vi "Evaluate Checksum.vi"(5 "Parallel in":refnum<class "Parallel.lvclass">, 6 "Path Builder":refnum<class "IPath Builder.lvclass">, 7 "Linked List ID":string, 8 "error in (no error)":errorcluster, 11 "Linked List Ref":refnum<data-value>) -> (0 "error out":errorcluster, 1 "Checksums Match":bool, 2 "Paths":path[](array[path]), 3 "Linked List Ref out":refnum<data-value>)   [LabVIEW 2017]
uses:
  linked-list/Source/Linked List/Linked List Ref/Linked List Ref.lvclass
  Parallel.lvclass
  linked-list/Source/Linked List/ILinkedList/ILinked List.lvclass
  Path Builder/IPath Builder/IPath Builder.lvclass
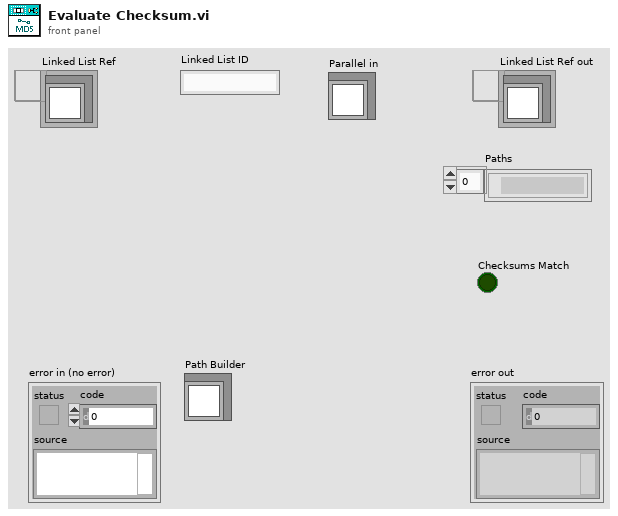
[diagram p1: front panel]
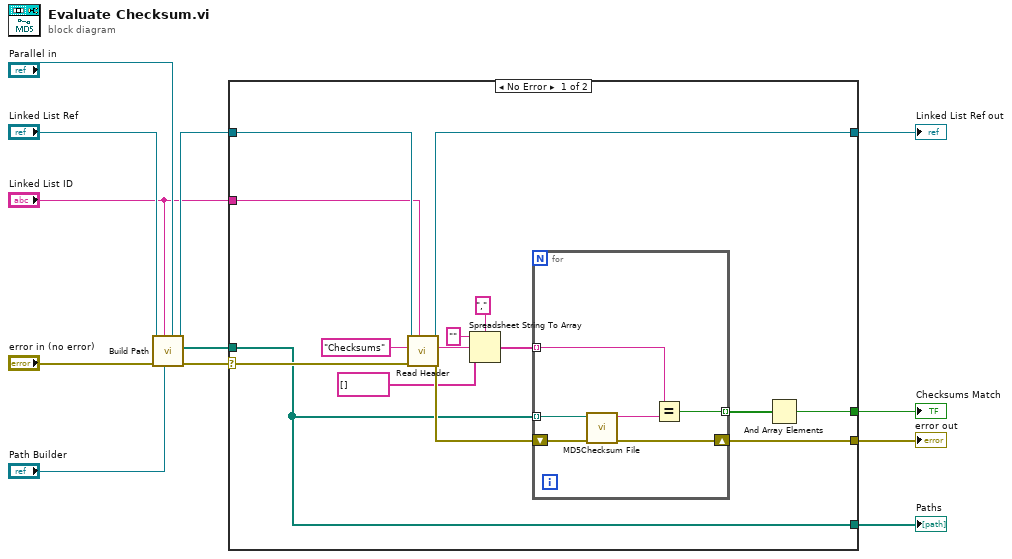
[diagram p0: block diagram]
diagram:
  n1 = call-dynamic "Build Path.vi"("Parallel in"="Parallel in", "Path Builder"="Path Builder", "Linked List ID"="Linked List ID", "error in (no error)"="error in (no error)", "Linked List Ref"="Linked List Ref") -> ("error out"=w5:errorcluster, "Paths"=w4:path[], "Linked List Ref out"=w8:refnum<data-value>)  [unwired: 4 in]
  n2 = case shown="No Error" w5 {
    selector: w5 -> [w20 w34]
    tunnel: [w18 _] -> w2
    tunnel: [w25 w35] -> w7
    tunnel: [w23 w34] -> w3
    tunnel: w8 -> [w22 w35]
    tunnel: "Linked List ID" -> [w21 _]
    tunnel: w4 -> [w19 _]
    tunnel: [w19 _] -> w1
    frame No Error {
      n3 = call "Read Header.vi"("Linked List ID"=w21, "error in (no error)"=w20, "Header Name"="Checksums", "Linked List Ref"=w22) -> ("error out"=w24:errorcluster, "Header Value"=w17:string, "Linked List Ref out"=w25:refnum<data-value>)  [unwired: 4 in, 1 out]
      n4 = Spreadsheet String To Array(delimiter (Tab)=",", format string="", spreadsheet string=w17, array type (2D Dbl)=string[] []) -> (array=w14:string[])
      n5 = for {
        tunnel: [w32] -> w26 mode=indexing
        tunnel: w19 -> [w29] mode=indexing
        shift-right: [w30] -> w23
        shift-left: w24 -> [w31]
        tunnel: w14 -> [w28] mode=indexing
        n6 = call <vilib>:"MD5Checksum File.vi"("error in (no error)"=w31, "Path"=w29) -> ("error out"=w30:errorcluster, "MD5 message-digest"=w33:string)  [unwired: 8 in]
        n7 = Equal?(x=w28, y=w33) -> (x = y?=w32:bool)
      }
      n8 = And Array Elements(Boolean array=w26) -> (logical AND=w18:bool)
    }
    frame Error {
    }
  }
  "Linked List Ref out" <- w7
  "error out" <- w3
  "Checksums Match" <- w2
  "Paths" <- w1
